vi "Animacion1.vi"() -> ()   [LabVIEW 2017]
uses:
  <vilib>/picture/picture.llb/Draw True-Color Pixmap.vi
panel:
  in  "Donde?":cluster{"x":i16, "y":i16}
  out "Mundo2":picture
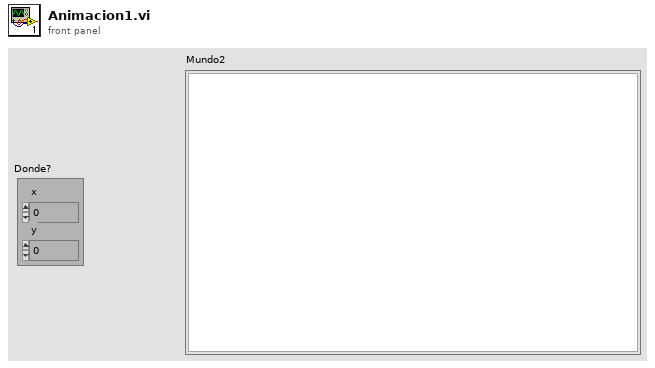
[diagram p1: front panel]
types:
  T1 = typedef "imagedata.ctl" = cluster{"image type":i32, "image depth":i32, "image":u8[], "mask":u8[], "colors":u32[], "Rectangle":cluster{"left":i16, "top":i16, "right":i16, "bottom":i16}}
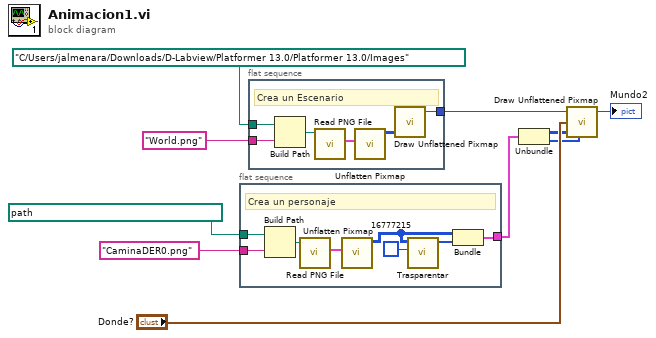
[diagram p0: block diagram]
diagram:
  n1 = flat-sequence {
    tunnel: path "F:/Prog/LabVIEW/Pruebas/Animación" ("path to PNG file") -> [w18]
    tunnel: "CaminaDER0.png" ("format string") -> [w17]
    tunnel: [w11] -> w3
    frame #0 {
      # "Crea un personaje"
      n2 = Build Path(base path=w18, name or relative path=w17) -> (appended path=w16:path)
      n3 = call <vilib>:"Read PNG File.vi"("path to PNG file"=w16) -> ("image data"=w15:T1)  [unwired: 8 in, 2 out]
      n4 = call <vilib>:"Unflatten Pixmap.vi"("image data"=w15) -> ("24-bit pixmap"=w13:u32[][])  [unwired: 4 in, 6 out]
      n5 = call "Trasparentar.vi"("Background Color"=u32 16777215, "24-bit pixmap"=w13) -> ("Mask"=w12:u8[])  [unwired: 9 in]
      n6 = Bundle("24-bit pixmap"=w13, "Mask"=w12) -> (w11:cluster{"24-bit pixmap":u32[][], "Mask":u8[]})  [unwired: 1 in]
    }
  }
  n7 = flat-sequence {
    tunnel: "World.png" ("format string") -> [w23]
    tunnel: path "C:/Users/jalmenara/Downloads/D-Labview/Platformer 13.0/Platformer 13.0/Images" ("path to PNG file") -> [w22]
    tunnel: [w19] -> w7
    frame #0 {
      # "Crea un Escenario"
      n8 = Build Path(base path=w22, name or relative path=w23) -> (appended path=w21:path)
      n9 = call <vilib>:"Read PNG File.vi"("path to PNG file"=w21) -> ("image data"=w24:T1)  [unwired: 8 in, 2 out]
      n10 = call <vilib>:"Unflatten Pixmap.vi"("image data"=w24) -> ("24-bit pixmap"=w20:u32[][])  [unwired: 4 in, 6 out]
      n11 = call-poly <vilib>:"Draw Unflattened Pixmap.vi"("data (RGB format)"=w20) -> ("new picture"=w19:picture)  [unwired: 8 in]
    }
  }
  n12 = Unbundle(w3) -> ("24-bit pixmap"=w2:u32[][], "Mask"=w1:u8[])
  n13 = call-poly <vilib>:"Draw Unflattened Pixmap.vi"("picture"=w7, "top left point(0, 0)"="Donde?", "data (RGB format)"=w2, "mask"=w1) -> ("new picture"=→"Mundo2":picture)  [unwired: 5 in]
